vi "DACDirect.vi"(7 "DeviceIndex":u32, 8 "error in (no error)":errorcluster) -> (0 "error out":errorcluster)   [LabVIEW 2011]
doc: "unsigned long CTR_8254ModeLoad(\nunsigned long DeviceIndex - number from 0-31 indicating on which device you wish to mode\nand load an 8254 counter\nunsigned long BlockIndex - number indicating which 8254 you wish to mode and load\nunsigned long CounterIndex - number from 0-2 indicating which counter on the specified 8254\nyou wish to mode and load\n18\nunsigned long Mode - a number from 0-5 specifying which 8254 mode you want the specified\ncounter to be\nunsigned short LoadValue - a number from 0 to 65535 which you wish loaded into the specified\ncounter\n)"
uses:
  AIOUSB.dll
panel:
  in  "channel":u32
  in  "count":u32=100
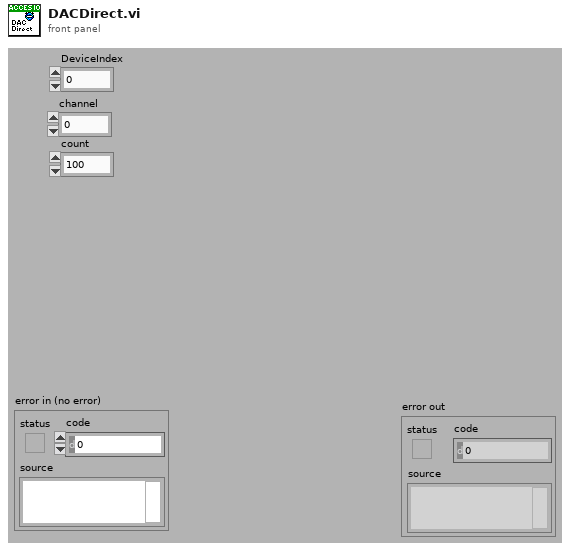
[diagram p1: front panel]
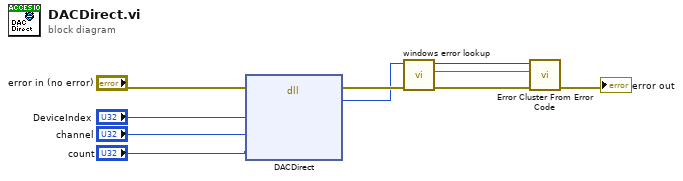
[diagram p0: block diagram]
diagram:
  n1 = dll-call lib="AIOUSB.dll" fn="DACDirect"(error in="error in (no error)", "DeviceIndex"="DeviceIndex", "channel"="channel", "counts"="count") -> (error out=w6:errorcluster, "return type"=w5:u32)  [unwired: 5 in, 1 out]
  n2 = call <instrlib>:"windows error lookup.vi"("error in (no error)"=w6, "Error Code"=w5) -> ("error out"=w8:errorcluster, "error message (\"\")"=w9:string)  [unwired: 8 in]
  n3 = call <vilib>:"Error Cluster From Error Code.vi"("error in (no error)"=w8, "error message (\"\")"=w9, "error code (0)"=w5) -> ("error out"=→"error out":errorcluster)  [unwired: 6 in]
